vi "LucaTest.vi"() -> ()   [LabVIEW 2009]
panel:
  in  "input cluster":T1={"left"=640, "right"=680, "top"=80, "bottom"=120}
  in  "Threshold":i32
  out "Intensity Graph":u16[][](graph)
  out "Counts":i32
  out "Ion":bool
  in  "stop":bool
  in  "Camera Index":i32=1
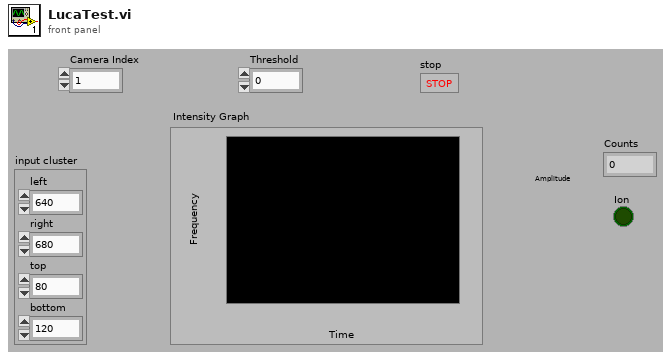
[diagram p1: front panel]
types:
  T1 = cluster{"left":i32, "right":i32, "top":i32, "bottom":i32}
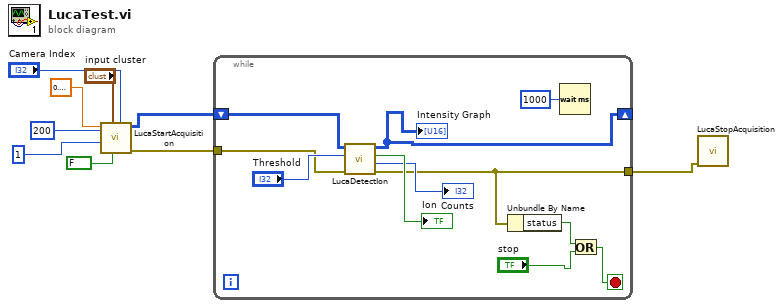
[diagram p0: block diagram]
diagram:
  n1 = call "LucaStartAcquisition.vi"("Camera Index"="Camera Index", "Continuous"=FALSE, "input cluster"="input cluster", "Bin Size"=1, "EMCCD Gain"=200, "Exposure Time"=sgl 0.3) -> ("error out"=w3:errorcluster, "Image"=w4:u16[][])  [unwired: 4 in]
  n2 = while {
    shift-right: [w17] -> _
    shift-left: w4 -> [w16]
    tunnel: w3 -> [w14]
    tunnel: [w13] -> w2
    stop <- w10 stop-if-true
    n3 = call "LucaDetectIon.vi"("error in (no error)"=w14, "Threshold"="Threshold", "array"=w16) -> ("error out"=w13:errorcluster, "Counts"=→"Counts":i32, "Ion"=→"Ion":bool, "output array"=w17:u16[][])  [unwired: 5 in]
    "Intensity Graph" <- w17
    n4 = Unbundle By Name(w13) -> ("status"=w11:bool)
    n5 = Wait (ms)(milliseconds to wait=u32 1000) -> ()  [unwired: 1 out]
    n6 = Or(x=w11, y="stop") -> (x .or. y?=w10:bool)
  }
  n7 = call "LucaStopAcquisition.vi"("error in (no error)"=w2) -> ()  [unwired: 10 in, 1 out]
